vi "Wheel Drawer.vi"(8 "error in":errorcluster, 11 "Data In":T1) -> (0 "error out":errorcluster, 3 "Data Out":T1)   [LabVIEW 2025]
uses:
  Controls/Wheel_data.ctl
  Controls/Spork plot.ctl
  Controls/Spoke_stats.ctl
  Controls/Spork type.ctl
  Controls/Tension.ctl
  Controls/Tension_Output.ctl
  Controls/Runout.ctl
  Controls/Runout Output.ctl
  Controls/Nippel Turn Direction.ctl
  Controls/Aditional Info.ctl
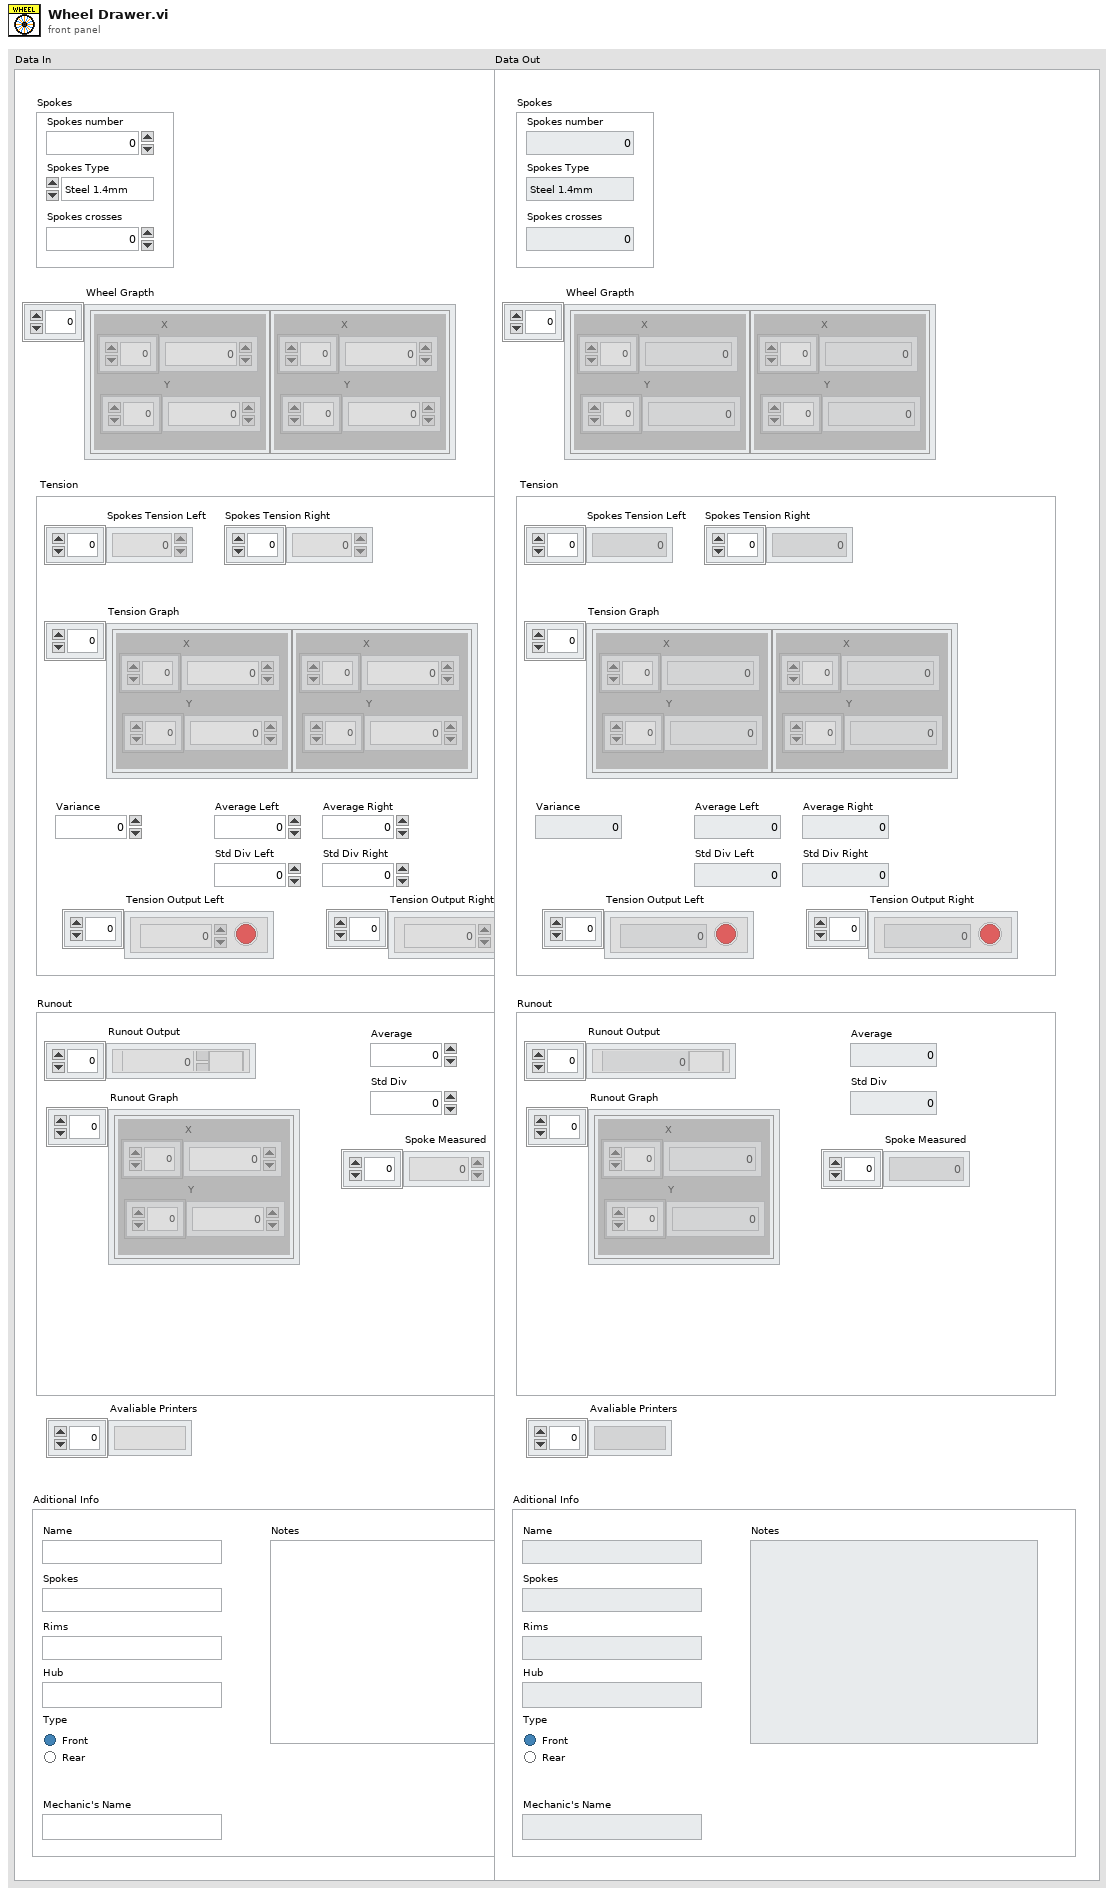
[diagram p1: front panel]
types:
  T1 = typedef "Wheel_data.ctl" = cluster{"Wheel Grapth":T2[], "Spokes":T3, "Tension":T5, "Runout":T7, "Avaliable Printers":string[], "Aditional Info":T10}
  T2 = typedef "Spork plot.ctl" = cluster{"X":dbl[], "Y":dbl[]}
  T3 = typedef "Spoke_stats.ctl" = cluster{"Spokes number":i32, "Spokes crosses":i32, "Spokes Type":T4}
  T4 = typedef "Spork type.ctl" = enum16{"Steel 1.4mm", "Steel 1.5mm", "Steel 1.6mm", "Steel 1.7mm", "Steel 1.8mm", "Steel 2mm", "Steel 2.3mm", "Steel 2.5mm", "Steel 2.6mm", "Aluminum 2.28mm", "Aluminum 2.54mm", "Aluminum 2.8mm", "Aluminum 3.3mm"}
  T5 = typedef "Tension.ctl" = cluster{"Spokes Tension Left":dbl[], "Tension Graph":T2[], "Average Left":dbl, "Variance":dbl, "Std Div Left":dbl, "Average Right":dbl, "Std Div Right":dbl, "Tension Output Left":T6[], "Tension Output Right":T6[], "Spokes Tension Right":dbl[]}
  T6 = typedef "Tension_Output.ctl" = cluster{"Tenction [kgf]":dbl, "Within Limit":bool}
  T7 = typedef "Runout.ctl" = cluster{"Runout Output":T8[], "Runout Graph":T2[], "Average":dbl, "Std Div":dbl, "Spoke Measured":i32[]}
  T8 = typedef "Runout Output.ctl" = cluster{"Value":dbl, "Nippel Direction":T9}
  T9 = typedef "Nippel Turn Direction.ctl" = u16
  T10 = typedef "Aditional Info.ctl" = cluster{"Name":string, "Rims":string, "Hub":string, "Notes":string, "Spokes":string, "Type":enum32{"Item 0", "Item 1"}, "Mechanic's Name":string}
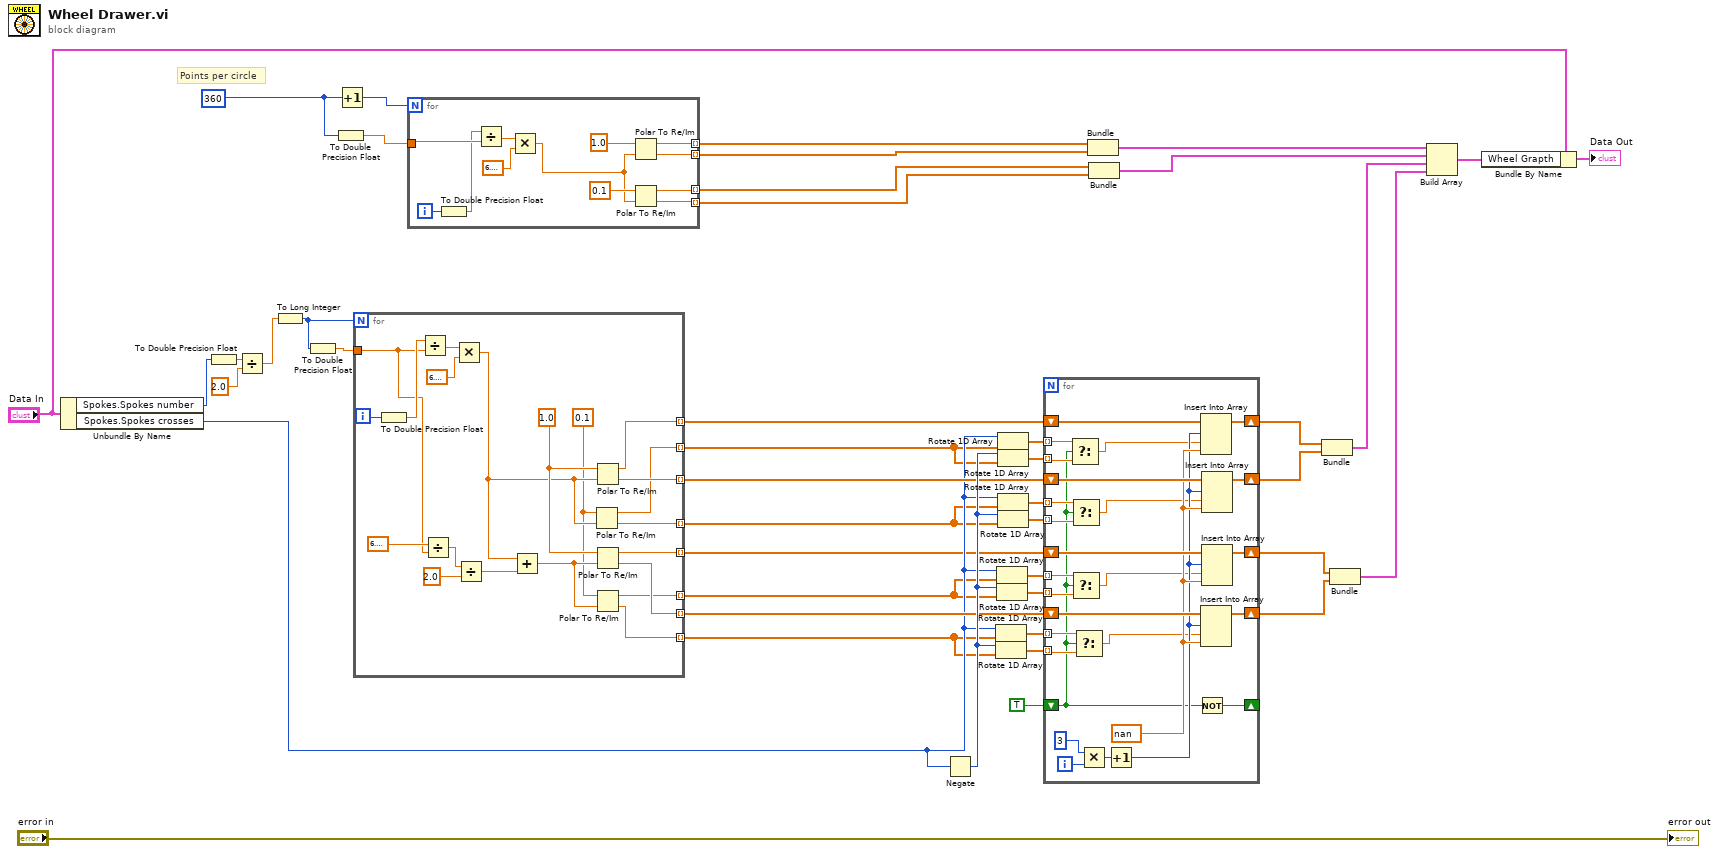
[diagram p0: block diagram]
diagram:
  w17 = 360
  # "Points per circle"
  n1 = Unbundle By Name("Data In") -> ("Spokes.Spokes number"=w9:i32, "Spokes.Spokes crosses"=w13:i32)
  n2 = To Double Precision Float(number=w9) -> (double precision float=w12:dbl)
  n3 = Divide(x=w12, y=2.0) -> (x/y=w10:dbl)
  n4 = To Long Integer(number=w10) -> (32bit integer=w11:i32)
  n5 = To Double Precision Float(number=w11) -> (double precision float=w40:dbl)
  n6 = To Double Precision Float(number=w17) -> (double precision float=w41:dbl)
  n7 = Increment(x=w17) -> (x+1=w42:i32)
  n8 = for {
    N: w11 -> [_]
    tunnel: w40 -> [w60]
    tunnel: [w56] -> w27 mode=indexing
    tunnel: [w55] -> w26 mode=indexing
    tunnel: [w54] -> w5 mode=indexing
    tunnel: [w53] -> w25 mode=indexing
    tunnel: [w48] -> w2 mode=indexing
    tunnel: [w47] -> w3 mode=indexing
    tunnel: [w46] -> w4 mode=indexing
    tunnel: [w45] -> w1 mode=indexing
    i -> [w63]
    w49 = 0.1 ("r")
    w52 = 1.0 ("r")
    n9 = To Double Precision Float(number=w63) -> (double precision float=w62:dbl)
    n10 = Divide(x=w62, y=w60) -> (x/y=w65:dbl)
    n11 = Divide(x=6.283185307179586, y=w60) -> (x/y=w58:dbl)
    n12 = Multiply(x=w65, y=6.283185307179586) -> (x*y=w51:dbl)
    n13 = Divide(x=w58, y=2.0) -> (x/y=w59:dbl)
    n14 = Add(x=w51, y=w59) -> (x+y=w50:dbl)
    n15 = Polar To Re/Im(2:w51, 3:w49) -> (0:w47:dbl, 1:w48:dbl)
    n16 = Polar To Re/Im(2:w51, 3:w52) -> (0:w55:dbl, 1:w56:dbl)
    n17 = Polar To Re/Im(2:w50, 3:w52) -> (0:w53:dbl, 1:w54:dbl)
    n18 = Polar To Re/Im(2:w50, 3:w49) -> (0:w45:dbl, 1:w46:dbl)
  }
  n19 = for {
    N: w42 -> [_]
    tunnel: w41 -> [w74]
    tunnel: [w71] -> w19 mode=indexing
    tunnel: [w72] -> w18 mode=indexing
    tunnel: [w67] -> w7 mode=indexing
    tunnel: [w66] -> w6 mode=indexing
    i -> [w77]
    n20 = To Double Precision Float(number=w77) -> (double precision float=w73:dbl)
    n21 = Divide(x=w73, y=w74) -> (x/y=w76:dbl)
    n22 = Multiply(x=w76, y=6.283185307179586) -> (x*y=w68:dbl)
    n23 = Polar To Re/Im(2:w68, 3:1.0 ("r")) -> (0:w71:dbl, 1:w72:dbl)
    n24 = Polar To Re/Im(2:w68, 3:0.1 ("r")) -> (0:w66:dbl, 1:w67:dbl)
  }
  n25 = Negate(x=w13) -> (-x=w30:i32)
  n26 = Rotate 1D Array(1:w1, 2:w13) -> (0:w34:dbl[])
  n27 = Rotate 1D Array(1:w1, 2:w30) -> (0:w31:dbl[])
  n28 = Rotate 1D Array(1:w4, 2:w13) -> (0:w35:dbl[])
  n29 = Rotate 1D Array(1:w4, 2:w30) -> (0:w29:dbl[])
  n30 = Rotate 1D Array(1:w2, 2:w13) -> (0:w37:dbl[])
  n31 = Rotate 1D Array(1:w2, 2:w30) -> (0:w33:dbl[])
  n32 = Rotate 1D Array(1:w3, 2:w13) -> (0:w36:dbl[])
  n33 = Rotate 1D Array(1:w3, 2:w30) -> (0:w32:dbl[])
  n34 = for {
    shift-right: [w103] -> w23
    shift-left: w27 -> [w104]
    shift-right: [w101] -> w24
    shift-left: w26 -> [w102]
    tunnel: w37 -> [w91] mode=indexing
    tunnel: w36 -> [w90] mode=indexing
    shift-right: [w96] -> w22
    shift-left: w5 -> [w97]
    shift-right: [w94] -> w21
    shift-left: w25 -> [w95]
    tunnel: w34 -> [w88] mode=indexing
    tunnel: w35 -> [w89] mode=indexing
    tunnel: w33 -> [w82] mode=indexing
    tunnel: w32 -> [w83] mode=indexing
    tunnel: w31 -> [w80] mode=indexing
    tunnel: w29 -> [w81] mode=indexing
    shift-right: [w79] -> _
    shift-left: TRUE -> [w78]
    i -> [w100]
    w93 = nan
    n35 = Select(t=w91, s=w78, f=w82) -> (s? t:f=w84:dbl)
    n36 = Select(t=w90, s=w78, f=w83) -> (s? t:f=w85:dbl)
    n37 = Select(t=w89, s=w78, f=w81) -> (s? t:f=w86:dbl)
    n38 = Select(t=w88, s=w78, f=w80) -> (s? t:f=w87:dbl)
    n39 = Multiply(x=3, y=w100) -> (x*y=w98:i32)
    n40 = Increment(x=w98) -> (x+1=w92:i32)
    n41 = Not(x=w78) -> (.not. x?=w79:bool)
    n42 = Insert Into Array(array=w104, index=w92, new element #1=w84, new element #2=w93) -> (w103:dbl[])
    n43 = Insert Into Array(array=w95, index=w92, new element #1=w87, new element #2=w93) -> (w94:dbl[])
    n44 = Insert Into Array(array=w102, index=w92, new element #1=w85, new element #2=w93) -> (w101:dbl[])
    n45 = Insert Into Array(array=w97, index=w92, new element #1=w86, new element #2=w93) -> (w96:dbl[])
  }
  n46 = Bundle(w18, w19) -> (w44:cluster{dbl[], dbl[]})  [unwired: 1 in]
  n47 = Bundle(w7, w6) -> (w43:cluster{dbl[], dbl[]})  [unwired: 1 in]
  n48 = Bundle(w23, w24) -> (w39:cluster{dbl[], dbl[]})  [unwired: 1 in]
  n49 = Bundle(w22, w21) -> (w38:cluster{dbl[], dbl[]})  [unwired: 1 in]
  n50 = Build Array(w44, w43, w39, w38) -> (w14:cluster{dbl[], dbl[]}[])
  n51 = Bundle By Name(cluster="Data In", "Wheel Grapth"=w14) -> (→"Data Out":T1)
  "error out" <- "error in"
